vi "save_infos.vi"() -> ()   [LabVIEW 2013]
panel:
  in  "Version":string="f"
  in  "Camera Serial":string="f"
  in  "Camera Model":string="f"
  in  "SOFT_VERSION":string="V2"
  in  "info Directory":path=path "D:/CONFIGS_TIME_LAPSE"
  in  "USED_FILTERS":u8[](array[numeric])
  in  "USED_LEDS":bool[][](array[boolean])=[[FALSE, FALSE], [TRUE, TRUE]]
  in  "Nstart":u32=30 step=1
  in  "Non":u32=150 step=1
  in  "Noff":u32 step=1
  in  "BETWEEN_PAT":u32
  in  "NPAT":u32
  in  "BETWEEN_SCAN":u32
  in  "NSCAN":u32
  in  "STAGE_PORT":refnum<visa-resource-name>="COM1"
  in  "STAGE_SPEED":dbl
  in  "ROMODE":u32
  in  "BIN":u16
  in  "EXPT":dbl
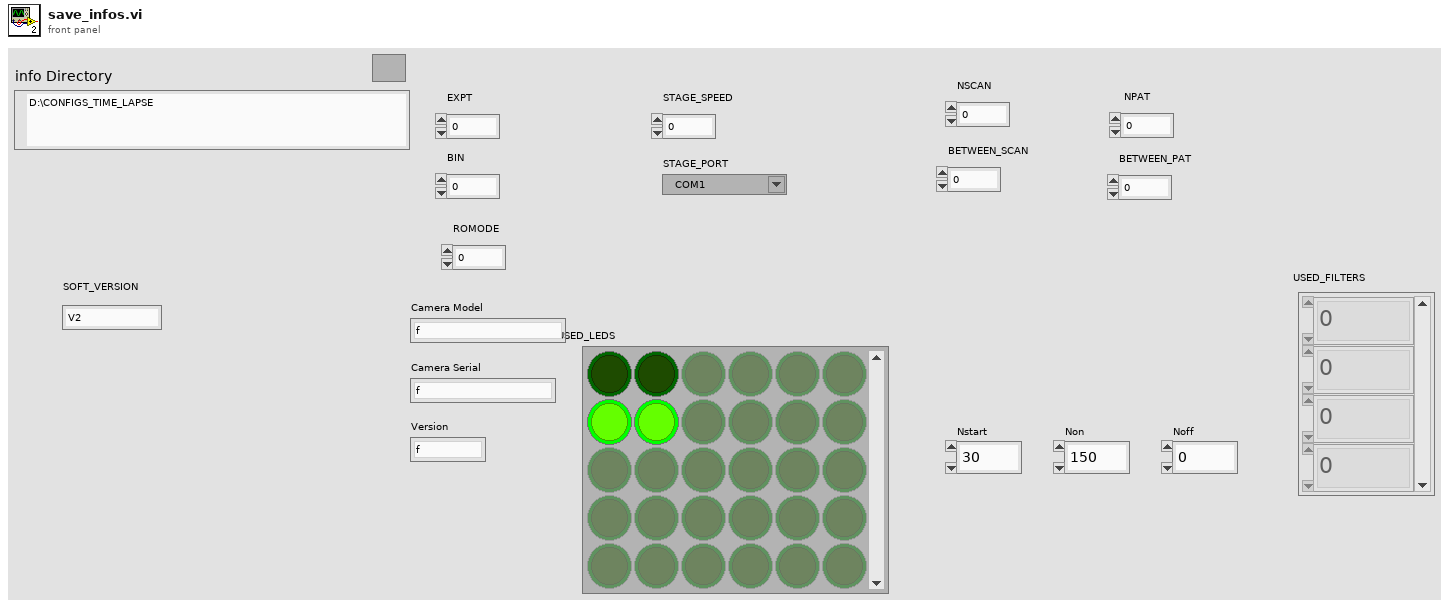
[diagram p1: front panel]
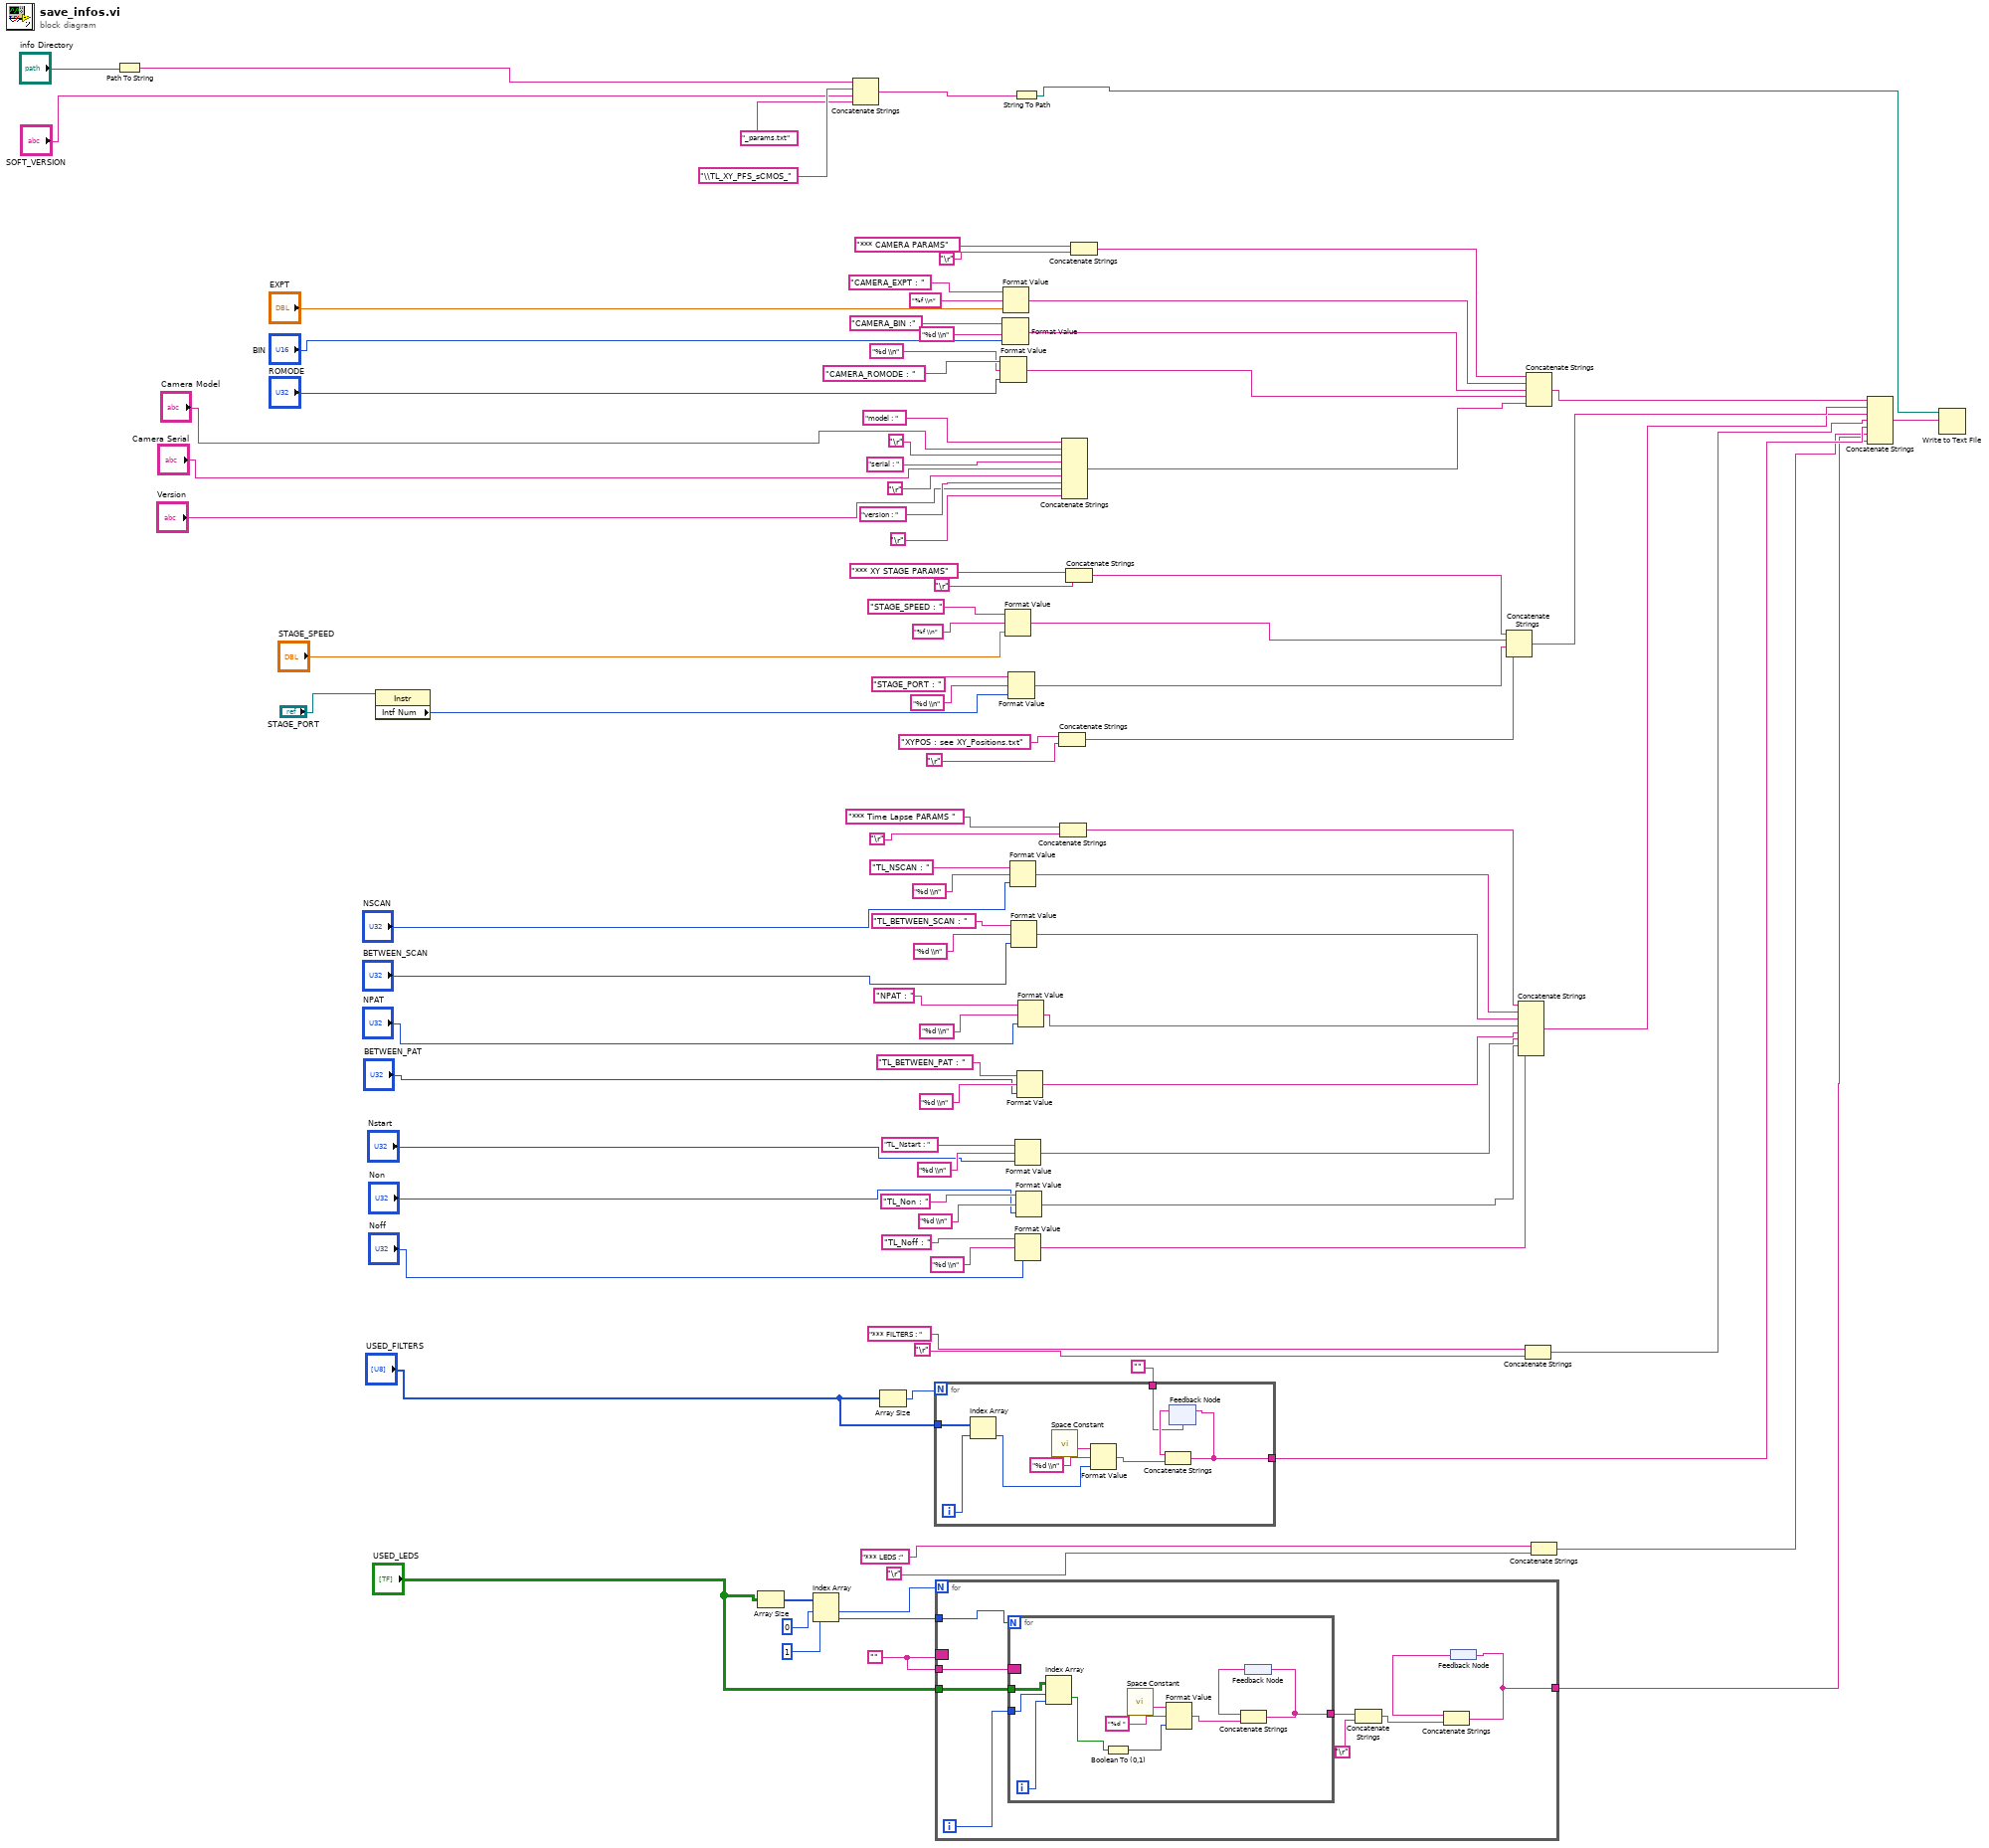
[diagram p0: block diagram]
diagram:
  w1 = ""
  n1 = Path To String(path="info Directory") -> (string=w99:string)
  n2 = property class="Instr"(reference="STAGE_PORT") -> ("Intf Num"=w74:u16)  [unwired: 1 in, 2 out]
  n3 = Array Size(array="USED_LEDS") -> (size(s)=w35:i32[])
  n4 = Index Array(array=w35, index #1=0, index #2=1) -> (element #1=w34:i32, element #2=w2:i32)
  n5 = Concatenate Strings(w99, "\\TL_XY_PFS_sCMOS_", "SOFT_VERSION", "_params.txt") -> (w95:string)
  n6 = Array Size(array="USED_FILTERS") -> (size(s)=w40:i32)
  n7 = for {
    N: w40 -> [_]
    tunnel: "USED_FILTERS" -> [w106]
    tunnel: "" -> [w102]
    tunnel: [w101] -> w11
    i -> [w107]
    n8 = Index Array(array=w106, index=w107) -> (element=w105:u8)
    n9 = call <vilib>:"Space Constant.vi"() -> ("String"=w108:string)
    n10 = Format Value(string ("")=w108, format string="%d \\n", value (0)=w105) -> (output string=w104:string)
    n11 = feedback #1(w102) -> (w103:string)
    n12 = Concatenate Strings(w103, w104) -> (w101:string)
    n13 = feedback-in #1(w101) -> ()
  }
  n14 = for {
    N: w34 -> [_]
    tunnel: "USED_LEDS" -> [w118]
    tunnel: [w112] -> w9
    tunnel: w2 -> [w111]
    border: w1 -> [_]
    tunnel: w1 -> [w110]
    i -> [w117]
    n15 = for {
      N: w111 -> [_]
      tunnel: w118 -> [w127]
      tunnel: w117 -> [w119]
      tunnel: [w121] -> w115
      border: w110 -> [_]
      i -> [w120]
      n16 = Index Array(array=w127, index (row)=w119, index (col)=w120) -> (element=w125:bool)
      n17 = Boolean To (0,1)(Boolean=w125) -> (0, 1=w124:i16)
      n18 = call <vilib>:"Space Constant.vi"() -> ("String"=w126:string)
      n19 = Format Value(string ("")=w126, format string="%d ", value (0)=w124) -> (output string=w123:string)
      n20 = feedback #2() -> (w122:string)
      n21 = Concatenate Strings(w122, w123) -> (w121:string)
      n22 = feedback-in #2(w121) -> ()
    }
    n23 = Concatenate Strings(w115, "\r") -> (w114:string)
    n24 = feedback #3() -> (w113:string)
    n25 = Concatenate Strings(w113, w114) -> (w112:string)
    n26 = feedback-in #3(w112) -> ()
  }
  n27 = Format Value(string ("")="CAMERA_ROMODE : ", format string="%d \\n", value (0)="ROMODE") -> (output string=w17:string)
  n28 = Format Value(string ("")="CAMERA_BIN :", format string="%d \\n", value (0)="BIN") -> (output string=w18:string)
  n29 = Format Value(string ("")="CAMERA_EXPT : ", format string="%f \\n", value (0)="EXPT") -> (output string=w19:string)
  n30 = Format Value(string ("")="STAGE_SPEED : ", format string="%f \\n", value (0)="STAGE_SPEED") -> (output string=w22:string)
  n31 = Format Value(string ("")="STAGE_PORT : ", format string="%d \\n", value (0)=w74) -> (output string=w21:string)
  n32 = Format Value(string ("")="TL_NSCAN : ", format string="%d \\n", value (0)="NSCAN") -> (output string=w30:string)
  n33 = Format Value(string ("")="TL_BETWEEN_SCAN : ", format string="%d \\n", value (0)="BETWEEN_SCAN") -> (output string=w29:string)
  n34 = String To Path(string=w95) -> (path=w7:path)
  n35 = Format Value(string ("")="TL_Nstart : ", format string="%d \\n", value (0)="Nstart") -> (output string=w26:string)
  n36 = Format Value(string ("")="TL_Noff : ", format string="%d \\n", value (0)="Noff") -> (output string=w24:string)
  n37 = Format Value(string ("")="TL_Non : ", format string="%d \\n", value (0)="Non") -> (output string=w25:string)
  n38 = Format Value(string ("")="TL_BETWEEN_PAT : ", format string="%d \\n", value (0)="BETWEEN_PAT") -> (output string=w27:string)
  n39 = Format Value(string ("")="NPAT : ", format string="%d \\n", value (0)="NPAT") -> (output string=w28:string)
  n40 = Concatenate Strings("XYPOS : see XY_Positions.txt", "\r") -> (w4:string)
  n41 = Concatenate Strings("*** Time Lapse PARAMS ", "\r") -> (w31:string)
  n42 = Concatenate Strings("model : ", "Camera Model", "\r", "serial : ", "Camera Serial", "\r", "version : ", "Version", "\r") -> (w16:string)
  n43 = Concatenate Strings("*** XY STAGE PARAMS", "\r") -> (w23:string)
  n44 = Concatenate Strings("*** CAMERA PARAMS", "\r") -> (w20:string)
  n45 = Concatenate Strings(w23, w22, w21, w4) -> (w14:string)
  n46 = Concatenate Strings(w31, w30, w29, w28, w27, w26, w25, w24) -> (w13:string)
  n47 = Concatenate Strings("*** FILTERS : ", "\r") -> (w12:string)
  n48 = Concatenate Strings(w20, w19, w18, w17, w16) -> (w15:string)
  n49 = Concatenate Strings("*** LEDS :", "\r") -> (w10:string)
  n50 = Concatenate Strings(w15, w14, w13, w12, w11, w10, w9) -> (w8:string)
  n51 = Write to Text File(file (use dialog)=w7, text=w8) -> ()  [unwired: 2 in, 3 out]
